vi "Finish Array Merge.vi"(8 "Array to Finish Index":i32, 9 "Array to Finish":cluster{"Key":string, "Value":variant}[](array[cluster]), 10 "Result Index in":i32, 11 "Result Array in":cluster{"Key":string, "Value":variant}[](array[cluster])) -> (2 "Result Index out":i32, 3 "Result Array out":cluster{"Key":string, "Value":variant}[](array[cluster]))   [LabVIEW 2020, in "UI Common.lvlib"]
uses:
  UI Common.lvlib
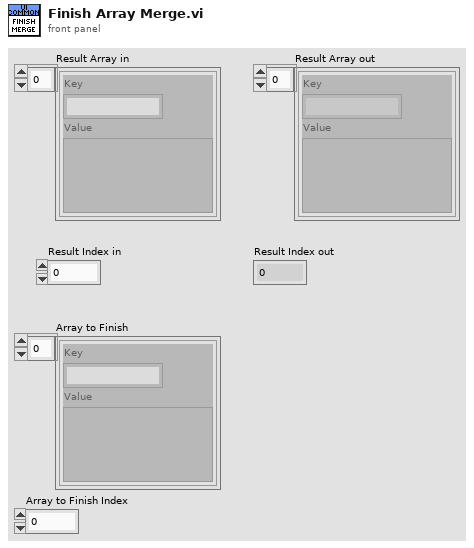
[diagram p1: front panel]
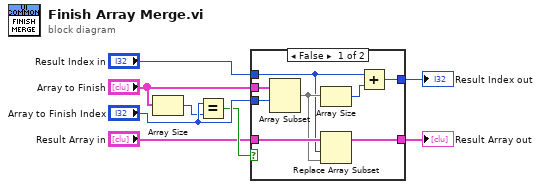
[diagram p0: block diagram]
diagram:
  n1 = Array Size(array="Array to Finish") -> (size(s)=w1:i32)
  n2 = Equal?(x="Array to Finish Index", y=w1) -> (x = y?=w7:bool)
  n3 = case shown="False" w7 {
    tunnel: "Result Array in" -> [w16 w18]
    tunnel: "Array to Finish Index" -> [w13 _]
    tunnel: "Result Index in" -> [w11 w17]
    tunnel: "Array to Finish" -> [w15 _]
    tunnel: [w9 w18] -> w5
    tunnel: [w10 w17] -> w4
    frame False {
      n4 = Array Subset(array=w15, index=w13) -> (w14:cluster{"Key":string, "Value":variant}[])  [unwired: 1 in]
      n5 = Array Size(array=w14) -> (size(s)=w12:i32)
      n6 = Replace Array Subset(array=w16, new element=w14, index=w11) -> (w9:cluster{"Key":string, "Value":variant}[])
      n7 = Add(x=w11, y=w12) -> (x+y=w10:i32)
    }
    frame True {
    }
  }
  "Result Array out" <- w5
  "Result Index out" <- w4
